vi "Get Port Status Response.vi"(8 "error in (no error)":errorcluster, 11 "Cypress in":refnum<class "Cypress.lvclass">) -> (0 "error out":errorcluster, 2 "Response":string, 3 "Cypress out":refnum<class "Cypress.lvclass">)   [LabVIEW 2020, in "Cypress.lvclass"]
uses:
  Cypress.lvclass
  Abstract/Serial device/Serial device.lvclass
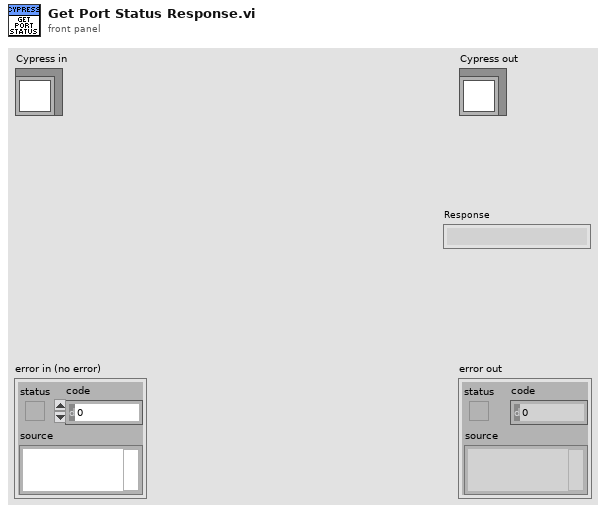
[diagram p1: front panel]
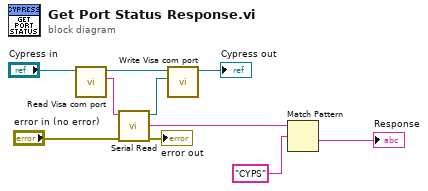
[diagram p0: block diagram]
diagram:
  n1 = call-dynamic "Read Visa com port.vi"("Serial device in"="Cypress in") -> ("Visa com port"=w10:string, "Serial device out"=w8:refnum<class "Cypress.lvclass">)  [unwired: 8 in, 1 out]
  n2 = call "Serial Read.vi"("error in (no error)"="error in (no error)", "VISA resource name in"=w10) -> ("error out"=→"error out":errorcluster, "Serial Response"=w2:string, "VISA resource name out"=w9:refnum<visa-resource-name>)  [unwired: 7 in]
  n3 = call-dynamic "Write Visa com port.vi"("Visa com port"=w9, "Serial device in"=w8) -> ("Serial device out"=→"Cypress out":refnum<class "Cypress.lvclass">)  [unwired: 8 in, 1 out]
  n4 = Match Pattern(string=w2, regular expression="CYPS") -> (after substring=→"Response":string)  [unwired: 1 in, 3 out]
